vi "Find Non-Overlapping Elf Claim.vi"(8 "error in (no error)":errorcluster, 10 "Trimmed Array":string[](array[string]), 11 "Fabric Claims":T1) -> (0 "error out":errorcluster, 3 "Non-Overlapping Elf Claim":i32)   [LabVIEW 2019]
uses:
  <vilib>/silver_ctls/ArrayMatrixCluster/Real Matrix NI_Silver.ctl
  <vilib>/Analysis/Matrix/Comparison/Equal/Equal - RM,RM.vi
  <vilib>/Analysis/Matrix/NI_Matrix.lvlib
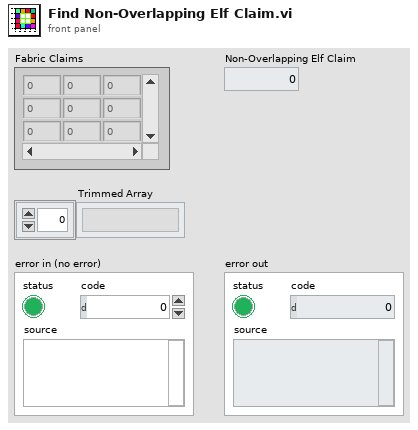
[diagram p1: front panel]
types:
  T1 = typedef "Real Matrix NI_Silver.ctl" = dbl[][]
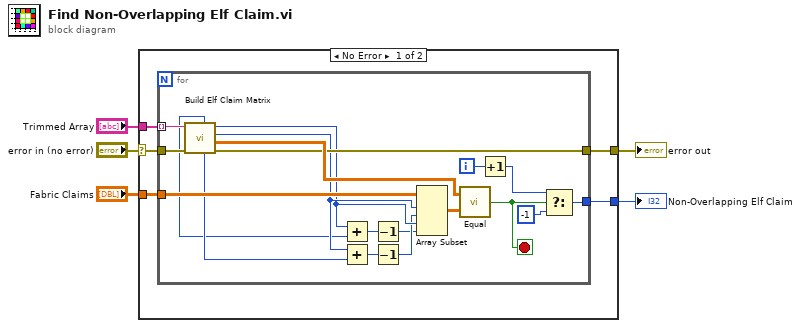
[diagram p0: block diagram]
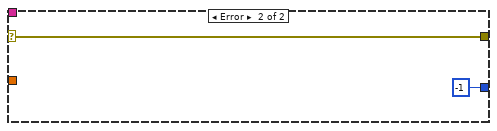
[diagram p2: hidden frame]
diagram:
  n1 = case shown="No Error" "error in (no error)" {
    selector: "error in (no error)" -> [w7 w31]
    tunnel: "Trimmed Array" -> [w10 _]
    tunnel: "Fabric Claims" -> [w9 _]
    tunnel: [w8 w31] -> w3
    tunnel: [w6 -1] -> w4
    frame No Error {
      n2 = for {
        tunnel: w10 -> [w29] mode=indexing
        tunnel: w9 -> [w28]
        tunnel: w7 -> [w25]
        tunnel: [w24] -> w8
        tunnel: [w21] -> w6
        i -> [w20]
        stop <- w23 stop-if-true
        n3 = call "Build Elf Claim Matrix.vi"("Error In"=w25, "Elf Claim"=w29) -> ("Error Out"=w24:errorcluster, "Elf Claim Matrix"=w26:T1, "Distance from Top Edge"=w18:i32, "Distance from Left Edge"=w16:i32, "Width of Claim"=w17:i32, "Height of Claim"=w15:i32)  [unwired: 4 in]
        n4 = Add(x=w16, y=w15) -> (x+y=w12:i32)
        n5 = Add(x=w18, y=w17) -> (x+y=w14:i32)
        n6 = Decrement(x=w12) -> (x-1=w11:i32)
        n7 = Decrement(x=w14) -> (x-1=w13:i32)
        n8 = Array Subset(array=w28, index (row)=w18, length (row)=w13, index (col)=w16, length (col)=w11) -> (w27:T1)
        n9 = call-poly <vilib>:"Equal.vi"("Real Matrix B"=w27, "Real Matrix A"=w26) -> ("A = B?"=w23:bool)
        n10 = Increment(x=w20) -> (x+1=w19:i32)
        n11 = Select(t=w19, s=w23, f=-1) -> (s? t:f=w21:i32)
      }
    }
    frame Error {
    }
  }
  "Non-Overlapping Elf Claim" <- w4
  "error out" <- w3
